vi "First Step.vi"(8 "error in (no error)":errorcluster, 11 "DAQ Digital Code Scan.lvclass in":refnum<class "DAQ Digital Code Scan.lvclass">) -> (0 "error out":errorcluster, 2 "Current Position":dbl, 3 "DAQ Digital Code Scan.lvclass out":refnum<class "DAQ Digital Code Scan.lvclass">)   [LabVIEW 2012, in "DAQ Digital Code Scan.lvclass"]
doc: "(Dynamic) Reset the instrument and prepare to scan. Go to step #0 - the first step. If desired, the scanner may do this in a different way than usual (i.e. by preparing to move a long distance, or reset to home position.)"
uses:
  DAQ Digital Code Scan.lvclass
  LabVIEW-programs/Scanners/Scanner/Scanner.lvclass
  DAQ Digital Code Scan.lvclass/DAQ Digital Code Scan.ctl
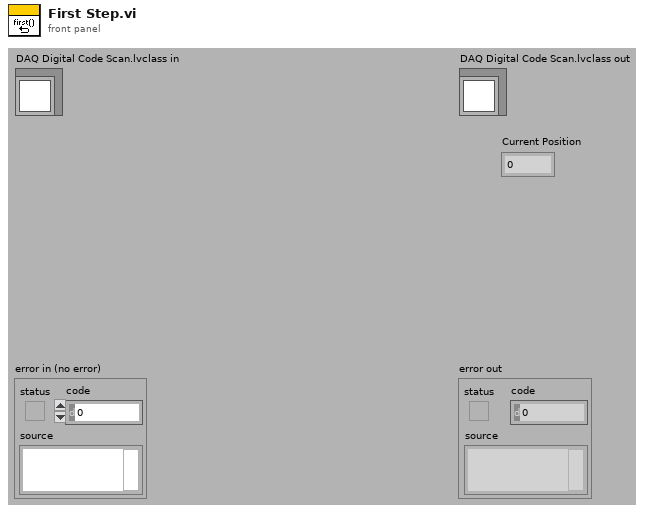
[diagram p1: front panel]
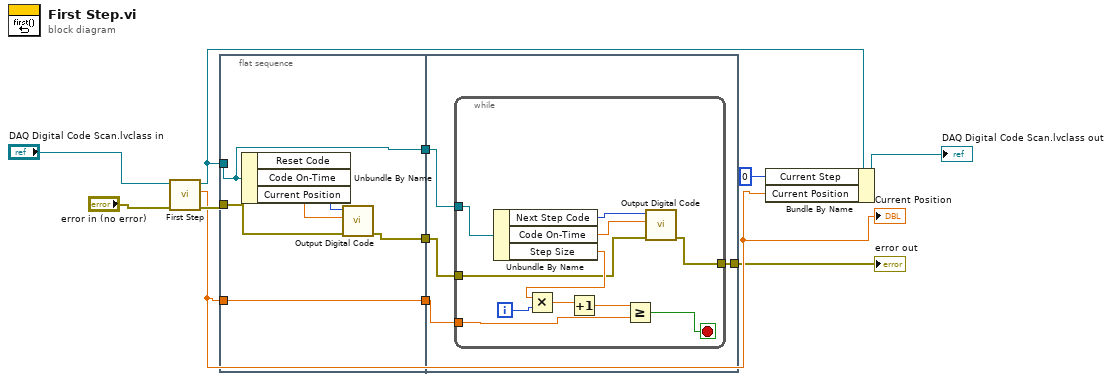
[diagram p0: block diagram]
diagram:
  n1 = call-parent "First Step.vi"("error in (no error)"="error in (no error)", "Scanner.lvclass in"="DAQ Digital Code Scan.lvclass in") -> ("error out"=w9:errorcluster, "Current Position"=w7:dbl, "Scanner.lvclass out"=w3:refnum<class "DAQ Digital Code Scan.lvclass">)  [unwired: 7 in]
  "Current Position" <- w7
  n2 = flat-sequence {
    tunnel: w3 -> [w12]
    tunnel: w9 -> [w15]
    tunnel: w7 -> [w14]
    tunnel: [w14] -> w6
    tunnel: [w13] -> w5
    tunnel: [w12] -> w2
    tunnel: w6 -> [w21]
    tunnel: w5 -> [w19]
    tunnel: w2 -> [w20]
    tunnel: [w18] -> w1
    frame #0 {
      n3 = Unbundle By Name(w12) -> ("Reset Code"=w17:i8, "Code On-Time"=w16:dbl)  [unwired: 1 out]
      n4 = call "Output Digital Code.vi"("error in (no error)"=w15, "Pulse Time"=w16, "Input"=w17) -> ("error out"=w13:errorcluster)  [unwired: 6 in]
    }
    frame #1 {
      n5 = while {
        tunnel: w21 -> [w31]
        tunnel: w20 -> [w29]
        tunnel: w19 -> [w25]
        tunnel: [w24] -> w18
        i -> [w32]
        stop <- w30 stop-if-true
        n6 = Unbundle By Name(w29) -> ("Next Step Code"=w28:i8, "Code On-Time"=w27:dbl, "Step Size"=w26:dbl)
        n7 = Multiply(x=w26, y=w32) -> (x*y=w23:dbl)
        n8 = Increment(x=w23) -> (x+1=w22:dbl)
        n9 = Greater Or Equal?(x=w22, y=w31) -> (x >= y?=w30:bool)
        n10 = call "Output Digital Code.vi"("error in (no error)"=w25, "Pulse Time"=w27, "Input"=w28) -> ("error out"=w24:errorcluster)  [unwired: 6 in]
      }
    }
  }
  n11 = Bundle By Name(cluster=w3, "Current Step"=u32 0, "Current Position"=w7) -> (→"DAQ Digital Code Scan.lvclass out":refnum<class "DAQ Digital Code Scan.lvclass">)
  "error out" <- w1
